vi "Trial - Save or Load.vi"(6 "Saving recipe to test directory?":bool, 7 "Trial Settings IN":T1={"Trial Label"="", "Type"="1.4", "Timeout (secs)"="", "Inter-Trial Interval (secs)"="", "Left Wall Enabled"=FALSE, "Right Wall Enabled"=FALSE, "Corridor Reset"=FALSE, "Default Wall Position"="", "Open Loop Change Positions"="", "Open Loop Values (mm)"="", "Corridor Width Change Positions"="", "Corridor Width Values (mm) "="", "Turn Change Positions"="0", "Turn Values (deg)"="1.4", "Left Texture Change Positions"="", "Right Texture Change Positions"="", "Video Frames (fps)"="", "Water Enabled"=FALSE, "Water Trial Position"="", "Photostimulation"="", "Water Corridor Max"="", "Water Range"="", "Water Drop Size (ms)"="", "Water Reward Position"="", "Duration (cm)"="", "Left Texture Enabled"=FALSE, "Right Texture Enabled"=FALSE, "Ps Trial Period"="", "Ps Inter-Pulse-Interval (ms)"="", "Ps Peak Power"="", "Ps Pulse Duration (ms)"="", "ephys_clock freq (hz)"="", "frame_clock (hz)"="", "Plot Color (Lateral Dist vs Trial Fraction)"=0}, 8 "Error IN":errorcluster, 10 "Trial Path IN":path, 11 "Command IN":T2) -> (0 "Error OUT":errorcluster, 3 "Trial Settings OUT":T1={"Trial Label"="", "Type"="1.4", "Timeout (secs)"="", "Inter-Trial Interval (secs)"="", "Left Wall Enabled"=FALSE, "Right Wall Enabled"=FALSE, "Corridor Reset"=FALSE, "Default Wall Position"="", "Open Loop Change Positions"="", "Open Loop Values (mm)"="", "Corridor Width Change Positions"="", "Corridor Width Values (mm) "="", "Turn Change Positions"="0", "Turn Values (deg)"="1.4", "Left Texture Change Positions"="", "Right Texture Change Positions"="", "Video Frames (fps)"="", "Water Enabled"=FALSE, "Water Trial Position"="", "Photostimulation"="", "Water Corridor Max"="", "Water Range"="", "Water Drop Size (ms)"="", "Water Reward Position"="", "Duration (cm)"="", "Left Texture Enabled"=FALSE, "Right Texture Enabled"=FALSE, "Ps Trial Period"="", "Ps Inter-Pulse-Interval (ms)"="", "Ps Peak Power"="", "Ps Pulse Duration (ms)"="", "ephys_clock freq (hz)"="", "frame_clock (hz)"="", "Plot Color (Lateral Dist vs Trial Fraction)"=0})   [LabVIEW 2018]
uses:
  controls/Command IN_Recipe.ctl
  controls/Trial Config Settings.ctl
  <vilib>/Utility/file.llb/Write Delimited Spreadsheet (string).vi
  <vilib>/Utility/file.llb/Read Delimited Spreadsheet (string).vi
  Globals/Global - Configuration Options.vi
panel:
  # "INPUTS"
  # "OUTPUTS"
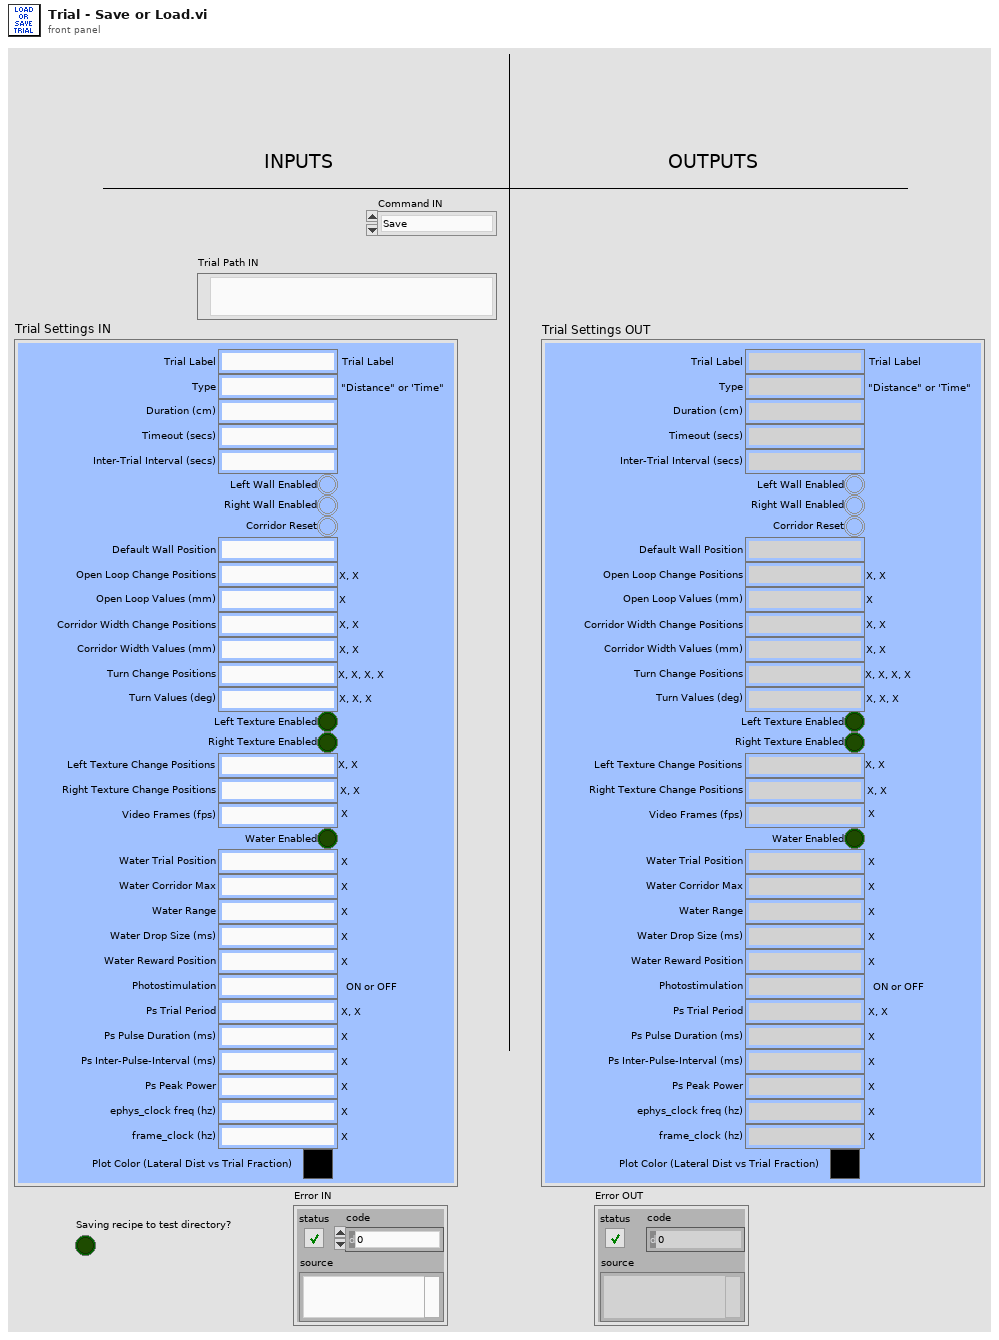
[diagram p1: front panel]
types:
  T1 = typedef "Trial Config Settings.ctl" = cluster{"Trial Label":string, "Type":string, "Timeout (secs)":string, "Inter-Trial Interval (secs)":string, "Left Wall Enabled":bool, "Right Wall Enabled":bool, "Corridor Reset":bool, "Default Wall Position":string, "Open Loop Change Positions":string, "Open Loop Values (mm)":string, "Corridor Width Change Positions":string, "Corridor Width Values (mm) ":string, "Turn Change Positions":string, "Turn Values (deg)":string, "Left Texture Change Positions":string, "Right Texture Change Positions":string, "Video Frames (fps)":string, "Water Enabled":bool, "Water Trial Position":string, "Photostimulation":string, "Water Corridor Max":string, "Water Range":string, "Water Drop Size (ms)":string, "Water Reward Position":string, "Duration (cm)":string, "Left Texture Enabled":bool, "Right Texture Enabled":bool, "Ps Trial Period":string, "Ps Inter-Pulse-Interval (ms)":string, "Ps Peak Power":string, "Ps Pulse Duration (ms)":string, "ephys_clock freq (hz)":string, "frame_clock (hz)":string, "Plot Color (Lateral Dist vs Trial Fraction)":u32}
  T2 = typedef "Command IN_Recipe.ctl" = enum16{"Save", "Load"}
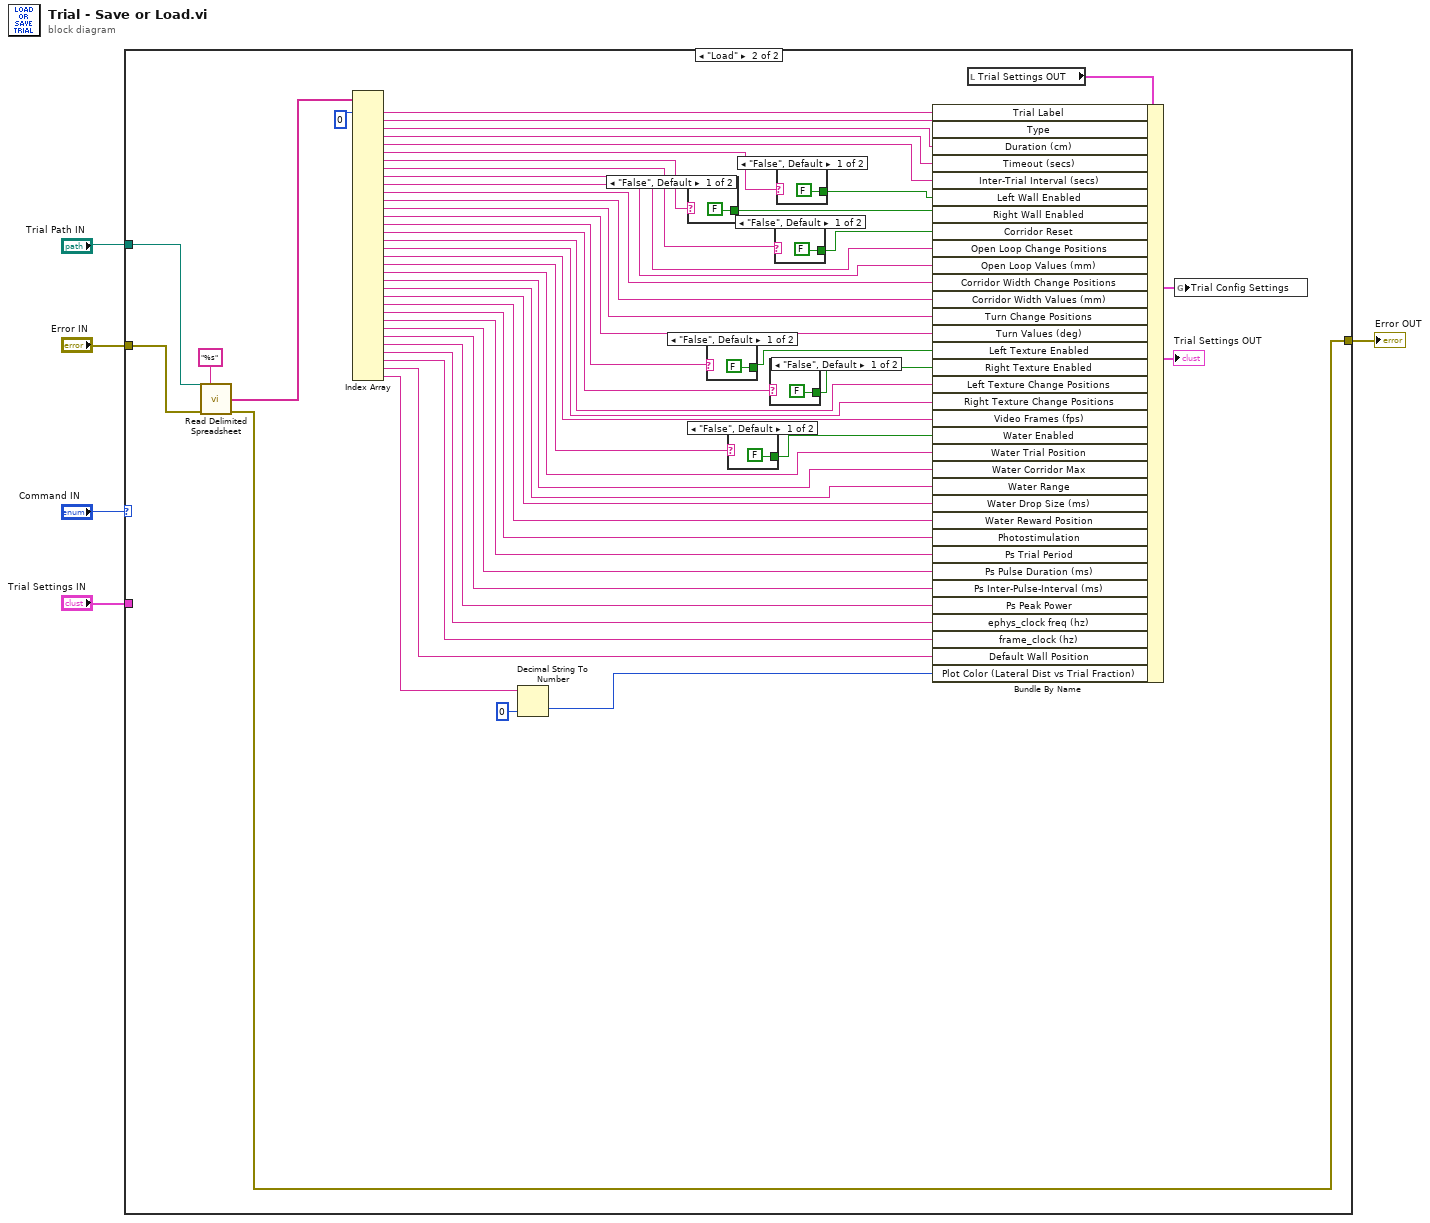
[diagram p0: block diagram]
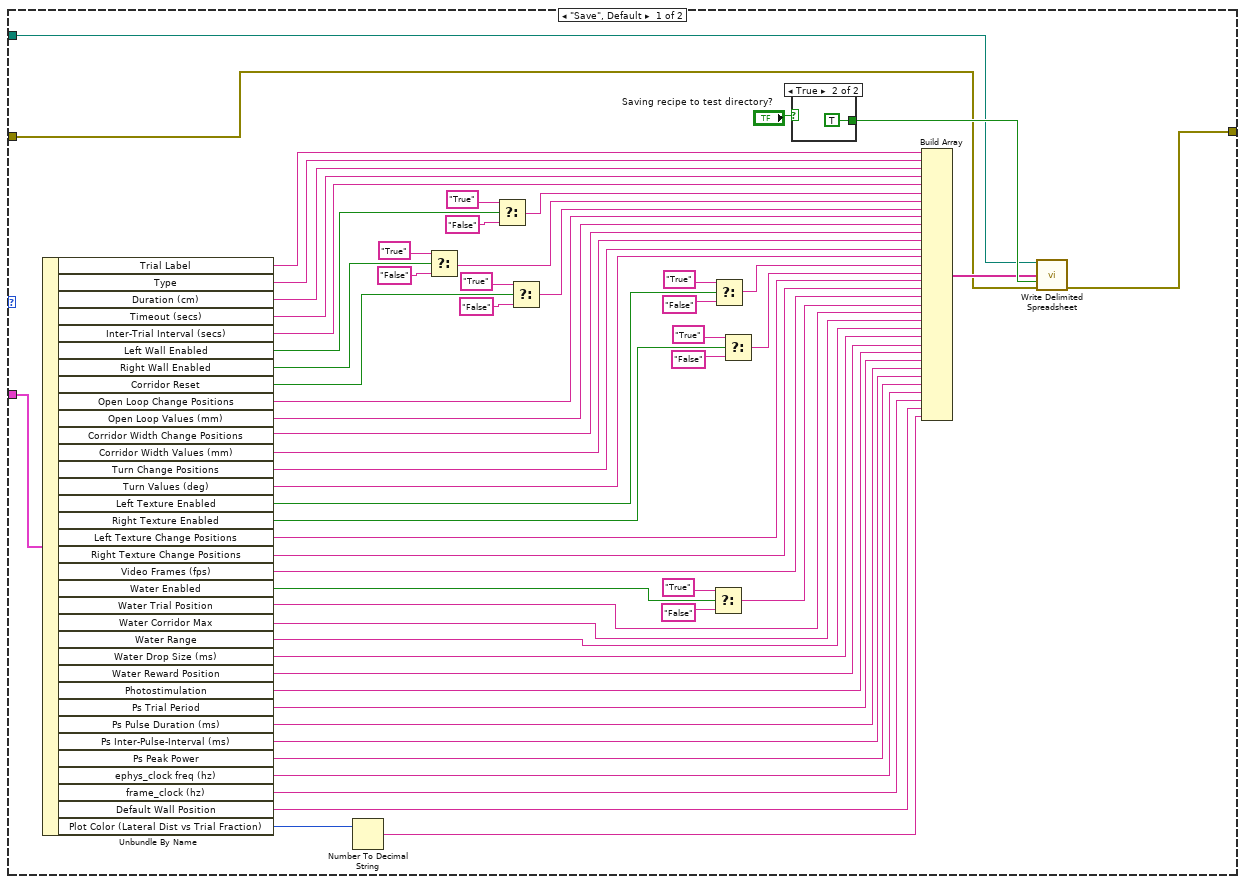
[diagram p2: hidden frame]
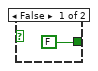
[diagram p3: hidden frame]
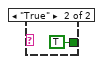
[diagram p4: hidden frame]
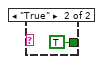
[diagram p5: hidden frame]
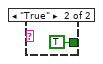
[diagram p6: hidden frame]
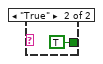
[diagram p7: hidden frame]
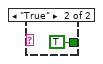
[diagram p8: hidden frame]
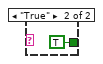
[diagram p9: hidden frame]
diagram:
  n1 = case shown="\"Load\"" "Command IN" {
    tunnel: "Trial Settings IN" -> [w65 _]
    tunnel: "Trial Path IN" -> [w63 w116]
    tunnel: [w61 w114] -> w5
    tunnel: "Error IN" -> [w60 w115]
    frame "Save", Default {
      n2 = Unbundle By Name(w65) -> ("Trial Label"=w34:string, "Type"=w58:string, "Duration (cm)"=w57:string, "Timeout (secs)"=w56:string, "Inter-Trial Interval (secs)"=w55:string, "Left Wall Enabled"=w52:bool, "Right Wall Enabled"=w44:bool, "Corridor Reset"=w43:bool, "Open Loop Change Positions"=w42:string, "Open Loop Values (mm)"=w41:string, "Corridor Width Change Positions"=w40:string, "Corridor Width Values (mm)"=w39:string, "Turn Change Positions"=w38:string, "Turn Values (deg)"=w37:string, "Left Texture Enabled"=w32:bool, "Right Texture Enabled"=w28:bool, "Left Texture Change Positions"=w27:string, "Right Texture Change Positions"=w26:string, "Video Frames (fps)"=w25:string, "Water Enabled"=w21:bool, "Water Trial Position"=w20:string, "Water Corridor Max"=w19:string, "Water Range"=w18:string, "Water Drop Size (ms)"=w17:string, "Water Reward Position"=w16:string, "Photostimulation"=w15:string, "Ps Trial Period"=w14:string, "Ps Pulse Duration (ms)"=w13:string, "Ps Inter-Pulse-Interval (ms)"=w12:string, "Ps Peak Power"=w11:string, "ephys_clock freq (hz)"=w10:string, "frame_clock (hz)"=w9:string, "Default Wall Position"=w8:string, "Plot Color (Lateral Dist vs Trial Fraction)"=w7:u32)
      n3 = Number To Decimal String(number=w7) -> (decimal integer string=w6:string)  [unwired: 1 in]
      n4 = Select(t="True", s=w44, f="False") -> (s? t:f=w46:string)
      n5 = Select(t="True", s=w52, f="False") -> (s? t:f=w51:string)
      n6 = Select(t="True", s=w43, f="False") -> (s? t:f=w45:string)
      n7 = Select(t="True", s=w21, f="False") -> (s? t:f=w22:string)
      n8 = Select(t="True", s=w32, f="False") -> (s? t:f=w33:string)
      n9 = Select(t="True", s=w28, f="False") -> (s? t:f=w29:string)
      n10 = case shown="True" "Saving recipe to test directory?" {
        tunnel: [FALSE ("append to file? (new file:F)") TRUE ("append to file? (new file:F)")] -> w64
        frame False {
        }
        frame True {
        }
      }
      n11 = Build Array(w34, w58, w57, w56, w55, w51, w46, w45, w42, w41, w40, w39, w38, w37, w33, w29, w27, w26, w25, w22, w20, w19, w18, w17, w16, w15, w14, w13, w12, w11, w10, w9, w8, w6) -> (w62:string[])
      n12 = call-poly <vilib>:"Write Delimited Spreadsheet.vi"("file path (dialog if empty)"=w63, "1D data"=w62, "append to file? (new file:F)"=w64, "error in (no error)"=w60) -> ("error out"=w61:errorcluster)  [unwired: 10 in, 1 out]
    }
    frame "Load" {
      n13 = call-poly <vilib>:"Read Delimited Spreadsheet.vi"("file path (dialog if empty)"=w116, "format (%s)"="%s" ("format (%.3f)"), "error in (no error)"=w115) -> ("first row"=w113:string[], "error out"=w114:errorcluster)  [unwired: 7 in, 4 out]
      n14 = Index Array(array=w113, index #1=0 ("index")) -> (element #1=w106:string, element #2=w105:string, element #3=w104:string, element #4=w103:string, element #5=w102:string, element #6=w112:string, element #7=w111:string, element #8=w110:string, element #9=w98:string, element #10=w97:string, element #11=w96:string, element #12=w95:string, element #13=w94:string, element #14=w93:string, element #15=w92:string, element #16=w91:string, element #17=w88:string, element #18=w87:string, element #19=w86:string, element #20=w84:string, element #21=w83:string, element #22=w82:string, element #23=w81:string, element #24=w80:string, element #25=w79:string, element #26=w78:string, element #27=w77:string, element #28=w76:string, element #29=w75:string, element #30=w74:string, element #31=w73:string, element #32=w72:string, element #33=w71:string, element #34=w70:string)  [unwired: 33 in]
      n15 = Decimal String To Number(string=w70, default (0L)=u32 0 ("default (0 I32)")) -> (number=w68:u32)  [unwired: 1 in, 1 out]
      n16 = case shown="\"False\", Default" w111 {
        tunnel: [FALSE TRUE] -> w100
        frame "False", Default {
        }
        frame "True" {
        }
      }
      n17 = case shown="\"False\", Default" w92 {
        tunnel: [FALSE TRUE] -> w90
        frame "False", Default {
        }
        frame "True" {
        }
      }
      n18 = case shown="\"False\", Default" w84 {
        tunnel: [FALSE TRUE] -> w85
        frame "False", Default {
        }
        frame "True" {
        }
      }
      n19 = case shown="\"False\", Default" w91 {
        tunnel: [FALSE TRUE] -> w89
        frame "False", Default {
        }
        frame "True" {
        }
      }
      n20 = case shown="\"False\", Default" w110 {
        tunnel: [FALSE TRUE] -> w99
        frame "False", Default {
        }
        frame "True" {
        }
      }
      n21 = case shown="\"False\", Default" w112 {
        tunnel: [FALSE TRUE] -> w101
        frame "False", Default {
        }
        frame "True" {
        }
      }
      n22 = local read "Trial Settings OUT"() -> (w108:T1)
      n23 = Bundle By Name(cluster=w108, "Trial Label"=w106, "Type"=w105, "Duration (cm)"=w104, "Timeout (secs)"=w103, "Inter-Trial Interval (secs)"=w102, "Left Wall Enabled"=w101, "Right Wall Enabled"=w100, "Corridor Reset"=w99, "Open Loop Change Positions"=w98, "Open Loop Values (mm)"=w97, "Corridor Width Change Positions"=w96, "Corridor Width Values (mm)"=w95, "Turn Change Positions"=w94, "Turn Values (deg)"=w93, "Left Texture Enabled"=w90, "Right Texture Enabled"=w89, "Left Texture Change Positions"=w88, "Right Texture Change Positions"=w87, "Video Frames (fps)"=w86, "Water Enabled"=w85, "Water Trial Position"=w83, "Water Corridor Max"=w82, "Water Range"=w81, "Water Drop Size (ms)"=w80, "Water Reward Position"=w79, "Photostimulation"=w78, "Ps Trial Period"=w77, "Ps Pulse Duration (ms)"=w76, "Ps Inter-Pulse-Interval (ms)"=w75, "Ps Peak Power"=w74, "ephys_clock freq (hz)"=w73, "frame_clock (hz)"=w72, "Default Wall Position"=w71, "Plot Color (Lateral Dist vs Trial Fraction)"=w68) -> (w107:T1)
      "Trial Settings OUT" <- w107
      n24 = global write "Global - Configuration Options.vi" "Trial Config Settings"(w107) -> ()
    }
  }
  "Error OUT" <- w5
